vi "Read ADC Volts.vi"(8 "error in (no error)":errorcluster, 10 "ADC Channel":T1, 11 "LINX-AutomationHat in":refnum<class "LINX-AutomationHat.lvclass">) -> (0 "error out":errorcluster, 2 "Value (V)":dbl, 3 "LINX-AutomationHat out":refnum<class "LINX-AutomationHat.lvclass">)   [LabVIEW 2020, in "LINX-AutomationHat.lvclass"]
doc: "Reads the automation-hats digital inputs."
uses:
  LINX-AutomationHat.lvclass
  ADC Channels.ctl
  LINX-ADS1015/Channel Selection.ctl
  LEDs.ctl
  LINX-ADS1015/LINX-ADS1X15.lvclass
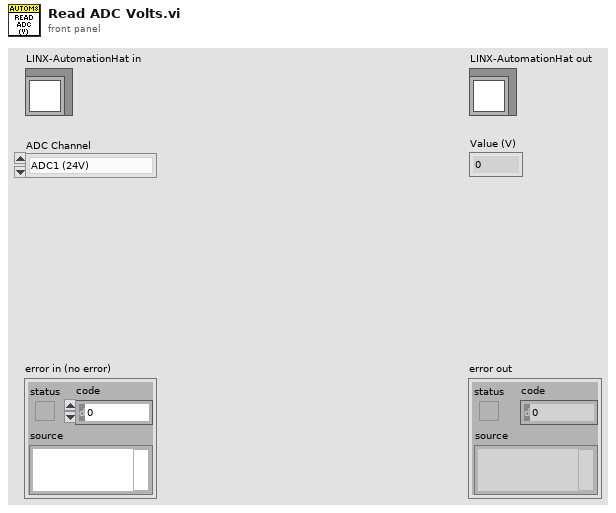
[diagram p1: front panel]
types:
  T1 = typedef "LINX-AutomationHat.lvclass/ADC Channels.ctl" = enum16{"ADC1 (24V)", "ADC2 (24V)", "ADC3 (24V)", "ADC4 (3.3v)"}
  T2 = typedef "LINX-AutomationHat.lvclass/LEDs.ctl" = enum16{"All", "ADC1", "ADC2", "ADC3", "Output1", "Output2", "Output3", "Relay1NO", "Relay1NC", "Relay2NO", "Relay2NC", "Relay3NO", "Relay3NC", "Input3", "Input2", "Input1", "Warn", "Comms", "Power"}
  T3 = typedef "LINX-ADS1X15.lvclass/Channel Selection.ctl" = u16
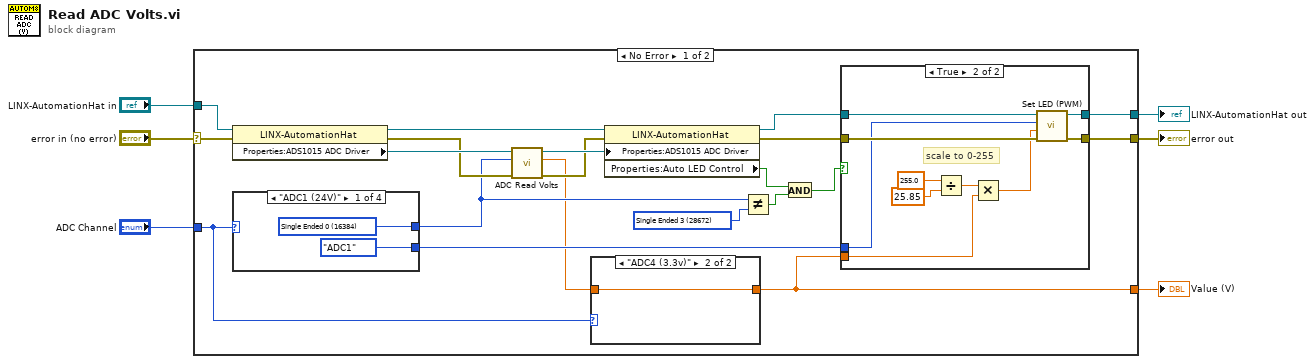
[diagram p0: block diagram]
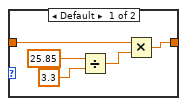
[diagram p2: hidden frame]
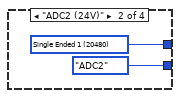
[diagram p3: hidden frame]
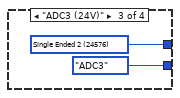
[diagram p4: hidden frame]
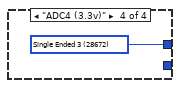
[diagram p5: hidden frame]
diagram:
  n1 = case shown="No Error" "error in (no error)" {
    selector: "error in (no error)" -> [w20 w53]
    tunnel: [w23 w53] -> w5
    tunnel: [w26 w52] -> w3
    tunnel: "LINX-AutomationHat in" -> [w22 w52]
    tunnel: "ADC Channel" -> [w8 _]
    tunnel: [w7 _] -> w1
    frame No Error {
      w11 = T3 28672 items=["Differential 0-1"=0, "Differential 2-3"=12288, "Single Ended 0"=16384, "Single Ended 1"=20480, "Single Ended 2"=24576, "Single Ended 3"=28672] ("y")
      n2 = property class="LINX-AutomationHat"(reference=w22, error in=w20) -> (reference out=w21:refnum<class "LINX-AutomationHat.lvclass">, error out=w17:errorcluster, "Properties:ADS1015 ADC Driver"=w19:refnum<class "LINX-ADS1X15.lvclass">)
      n3 = case shown="\"ADC1 (24V)\"" w8 {
        tunnel: [w34 w36 w38 w39] -> w12
        tunnel: [LEDs."ADC1" ("LED Selector") LEDs."ADC2" ("LED Selector") LEDs."ADC3" ("LED Selector") _] -> w15
        frame "ADC1 (24V)" {
          w34 = T3 16384 items=["Differential 0-1"=0, "Differential 2-3"=12288, "Single Ended 0"=16384, "Single Ended 1"=20480, "Single Ended 2"=24576, "Single Ended 3"=28672] ("ADC Channel Selection")
        }
        frame "ADC2 (24V)" {
          w36 = T3 20480 items=["Differential 0-1"=0, "Differential 2-3"=12288, "Single Ended 0"=16384, "Single Ended 1"=20480, "Single Ended 2"=24576, "Single Ended 3"=28672] ("ADC Channel Selection")
        }
        frame "ADC3 (24V)" {
          w38 = T3 24576 items=["Differential 0-1"=0, "Differential 2-3"=12288, "Single Ended 0"=16384, "Single Ended 1"=20480, "Single Ended 2"=24576, "Single Ended 3"=28672] ("ADC Channel Selection")
        }
        frame "ADC4 (3.3v)" {
          w39 = T3 28672 items=["Differential 0-1"=0, "Differential 2-3"=12288, "Single Ended 0"=16384, "Single Ended 1"=20480, "Single Ended 2"=24576, "Single Ended 3"=28672] ("ADC Channel Selection")
        }
      }
      n4 = call "ADC Read Volts.vi"("error in (no error)"=w17, "ADC Channel Selection"=w12, "LINX-ADS1X15 in"=w19) -> ("error out"=w16:errorcluster, "ADC Volts"=w9:dbl, "LINX-ADS1X15 out"=w18:refnum<class "LINX-ADS1X15.lvclass">)  [unwired: 6 in]
      n5 = case shown="\"ADC4 (3.3v)\"" w8 {
        tunnel: w9 -> [w28 w32]
        tunnel: [w27 w32] -> w7
        frame Default {
          n6 = Divide(x=25.85, y=3.3) -> (x/y=w29:dbl)
          n7 = Multiply(x=w28, y=w29) -> (x*y=w27:dbl)
        }
        frame "ADC4 (3.3v)" {
        }
      }
      n8 = property class="LINX-AutomationHat"(reference=w21, error in=w16, "Properties:ADS1015 ADC Driver"=w18) -> (reference out=w25:refnum<class "LINX-AutomationHat.lvclass">, error out=w24:errorcluster, "Properties:Auto LED Control"=w14:bool)
      n9 = Not Equal?(x=w12, y=w11) -> (x != y?=w10:bool)
      n10 = And(x=w14, y=w10) -> (x .and. y?=w13:bool)
      n11 = case shown="True" w13 {
        tunnel: [w41 w51] -> w26
        tunnel: w25 -> [w41 w50]
        tunnel: w24 -> [w40 w49]
        tunnel: [w40 w48] -> w23
        tunnel: w15 -> [_ w47]
        tunnel: w7 -> [_ w42]
        frame False {
        }
        frame True {
          # "scale to 0-255"
          n12 = Divide(x=255.0, y=25.85) -> (x/y=w44:dbl)
          n13 = Multiply(x=w44, y=w42) -> (x*y=w43:dbl)
          n14 = call-dynamic "Set LED (PWM).vi"("error in (no error)"=w49, "PWM (0-255)"=w43, "LED Selector"=w47, "LINX-AutomationHat in"=w50) -> ("error out"=w48:errorcluster, "LINX-AutomationHat out"=w51:refnum<class "LINX-AutomationHat.lvclass">)  [unwired: 6 in]
        }
      }
    }
    frame Error {
    }
  }
  "error out" <- w5
  "LINX-AutomationHat out" <- w3
  "Value (V)" <- w1
